vi "limitDecendantsTo1Level.vi"(8 "error in (no error)":errorcluster, 10 "hierarchy":string[][](array[string]), 11 "ClassLoader in":refnum<class "ClassLoader.lvclass">) -> (0 "error out":errorcluster, 2 "hierarchy out":string[][](array[string]), 3 "ClassLoader out":refnum<class "ClassLoader.lvclass">)   [LabVIEW 2020, in "JKI JSON Object Serialization.lvlib" / "OOP_Utility.lvlib" / "Reflection.lvclass"]
doc: "GCraftsman JSON Object Serialization Toolkit\nwww.GCraftsman.com\nCopyright (c) 2017, GCraftsman"
uses:
  Reflection.lvclass
  ClassLoader/ClassLoader.lvclass
  Reflection.lvclass/Reflection.ctl
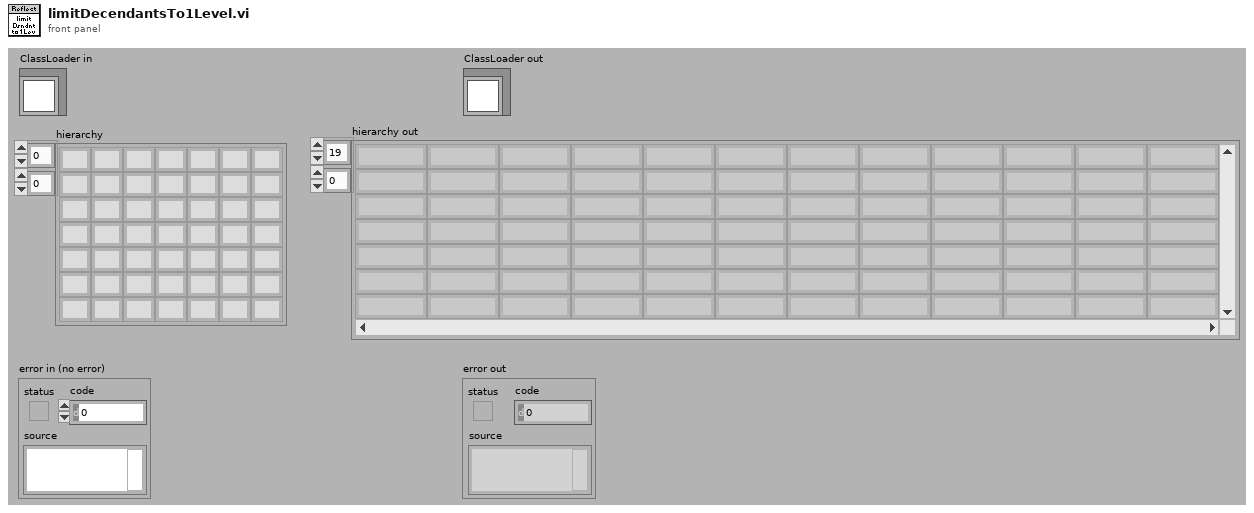
[diagram p1: front panel]
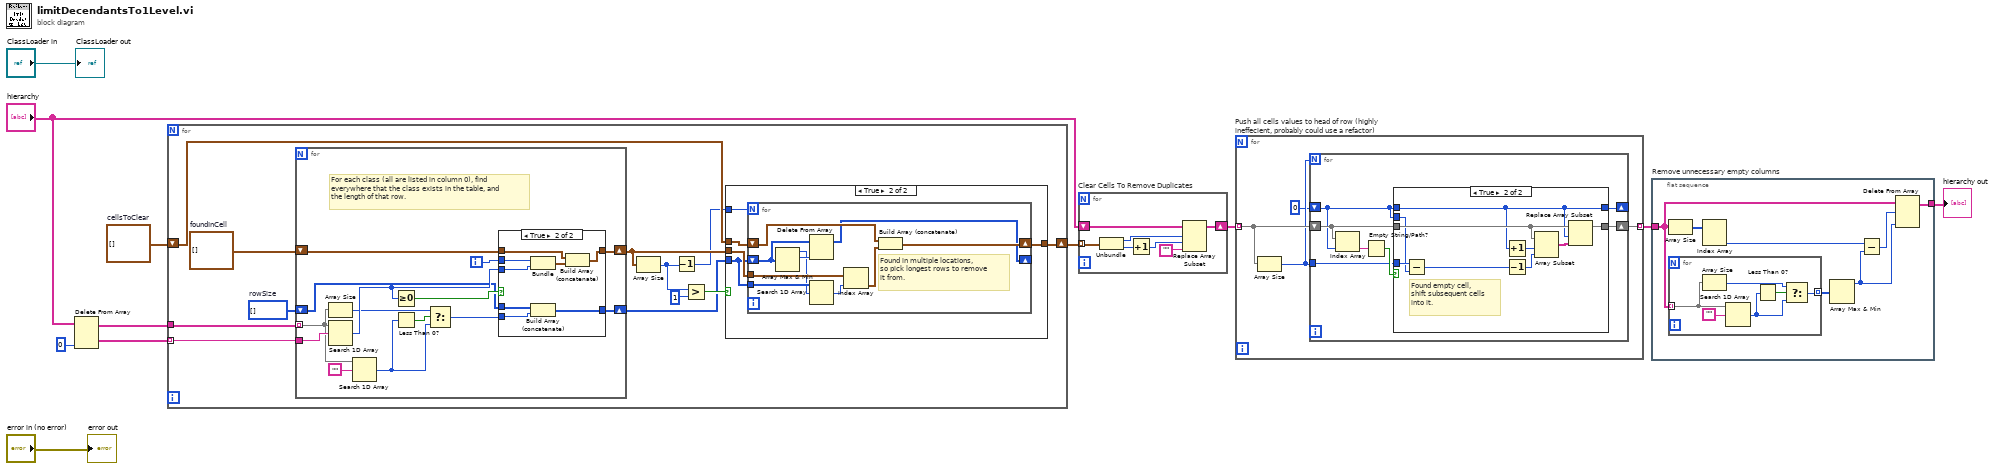
[diagram p0: block diagram]
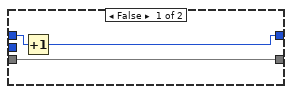
[diagram p2: hidden frame]
diagram:
  w8 = cluster{i32, "index of element":i32}[] []  # cellsToClear
  n1 = Delete From Array(array="hierarchy", index (col)=0 ("disabled index (col)")) -> (deleted portion=w4:string[], array with subset deleted=w5:string[][])  [unwired: 2 in]
  n2 = for {
    tunnel: w5 -> [w22]
    tunnel: w4 -> [w23] mode=indexing
    shift-right: [w15] -> w9
    shift-left: w8 -> [w14]
    w20 = i32[] []  # rowSize
    w21 = cluster{i32, "index of element":i32}[] []  # foundInCell
    n3 = for {
      tunnel: w23 -> [w52]
      tunnel: w22 -> [w43] mode=indexing
      shift-right: [w50] -> w16
      shift-left: w21 -> [w47]
      shift-right: [w46] -> w17
      shift-left: w20 -> [w45]
      i -> [w48]
      # "For each class (all are listed in column 0), find \neverywhere that the class exists in the table, and\nthe length of that row."
      n4 = Array Size(array=w43) -> (size(s)=w42:i32)
      n5 = Search 1D Array(1D array=w43, element=w52) -> (index of element=w49:i32)  [unwired: 1 in]
      n6 = Search 1D Array(1D array=w43, element="") -> (index of element=w41:i32)  [unwired: 1 in]
      n7 = Greater Or Equal To 0?(x=w49) -> (x >= 0?=w51:bool)
      n8 = Less Than 0?(x=w41) -> (x < 0?=w44:bool)
      n9 = Select(t=w42, s=w44, f=w41) -> (s? t:f=w40:i32)
      n10 = case shown="True" w51 {
        tunnel: w40 -> [_ w58]
        tunnel: [w55 w63] -> w50
        tunnel: w49 -> [_ w62]
        tunnel: w48 -> [_ w61]
        tunnel: w47 -> [w55 w59]
        tunnel: [w54 w57] -> w46
        tunnel: w45 -> [w54 w56]
        frame False {
        }
        frame True {
          n11 = Bundle(w61, "index of element"=w62) -> (w60:cluster{i32, "index of element":i32})  [unwired: 1 in]
          n12 = Build Array (concatenate)(w56, w58) -> (w57:i32[])
          n13 = Build Array (concatenate)(w59, w60) -> (w63:cluster{i32, "index of element":i32}[])
        }
      }
    }
    n14 = Array Size(array=w16) -> (size(s)=w13:i32)
    n15 = Decrement(x=w13) -> (x-1=w12:i32)
    n16 = Greater?(x=w13, y=1) -> (0:w18:bool)
    n17 = case shown="True" w18 {
      tunnel: w17 -> [_ w25]
      tunnel: w16 -> [_ w29]
      tunnel: [w24 w28] -> w15
      tunnel: w14 -> [w24 w27]
      tunnel: w12 -> [_ w26]
      frame False {
      }
      frame True {
        n18 = for {
          N: w26 -> [_]
          tunnel: w29 -> [w39]
          shift-right: [w37] -> w28
          shift-left: w27 -> [w36]
          shift-right: [w35] -> _
          shift-left: w25 -> [w32]
          tunnel: w25 -> [w33]
          # "Found in multiple locations,\nso pick longest rows to remove\nit from."
          n19 = Array Max & Min(array=w32) -> (max value=w31:i32, max index (indices)=w34:i32)  [unwired: 2 out]
          n20 = Delete From Array(array=w32, index=w34) -> (array with subset deleted=w35:i32[])  [unwired: 1 in, 1 out]
          n21 = Search 1D Array(1D array=w33, element=w31) -> (index of element=w30:i32)  [unwired: 1 in]
          n22 = Index Array(array=w39, index=w30) -> (element=w38:cluster{i32, "index of element":i32})
          n23 = Build Array (concatenate)(w36, w38) -> (w37:cluster{i32, "index of element":i32}[])
        }
      }
    }
  }
  n24 = for "Clear Cells To Remove Duplicates" {
    tunnel: w9 -> [w68] mode=indexing
    shift-right: [w64] -> w3
    shift-left: "hierarchy" -> [w70]
    n25 = Unbundle(w68) -> (w69:i32, "index of element"=w66:i32)
    n26 = Increment(x=w66) -> (x+1=w65:i32)
    n27 = Replace Array Subset(array=w70, new element="", index (row)=w69, index (col)=w65) -> (w64:string[][])
  }
  n28 = for "Push all cells values to head of row (highly ineffecient, probably could use a refactor)" {
    tunnel: w3 -> [w74] mode=indexing
    tunnel: [w73] -> w2 mode=indexing
    n29 = Array Size(array=w74) -> (size(s)=w72:i32)
    n30 = for {
      N: w72 -> [_]
      shift-right: [w78] -> w73
      shift-left: w74 -> [w80]
      tunnel: w72 -> [w76]
      shift-right: [w77] -> _
      shift-left: 0 -> [w75]
      n31 = Index Array(array=w80, index=w75) -> (element=w81:string)
      n32 = Empty String/Path?(string/path=w81) -> (empty?=w79:bool)
      n33 = case shown="True" w79 {
        tunnel: w80 -> [w84 w93]
        tunnel: w75 -> [w82 w85]
        tunnel: [w84 w91] -> w78
        tunnel: [w83 w85] -> w77
        tunnel: w76 -> [_ w89]
        tunnel: w75 -> [_ w88]
        frame False {
          n34 = Increment(x=w82) -> (x+1=w83:i32)
        }
        frame True {
          # "Found empty cell,\nshift subsequent cells\ninto it."
          n35 = Subtract(x=w89, y=w88) -> (x-y=w90:i32)
          n36 = Increment(x=w85) -> (x+1=w86:i32)
          n37 = Decrement(x=w90) -> (x-1=w87:i32)
          n38 = Array Subset(array=w93, index=w86, length=w87) -> (w92:string[])
          n39 = Replace Array Subset(array=w93, new element=w92, index=w85) -> (w91:string[])
        }
      }
    }
  }
  n40 = flat-sequence "Remove unnecessary empty columns" {
    tunnel: w2 -> [w99]
    tunnel: [w95] -> w1
    frame #0 {
      n41 = Array Size(array=w99) -> (size(s)=w98:i32[])
      n42 = for {
        tunnel: w99 -> [w103] mode=indexing
        tunnel: [w102] -> w100 mode=indexing
        n43 = Array Size(array=w103) -> (size(s)=w104:i32)
        n44 = Search 1D Array(1D array=w103, element="") -> (index of element=w101:i32)  [unwired: 1 in]
        n45 = Less Than 0?(x=w101) -> (x < 0?=w105:bool)
        n46 = Select(t=w104, s=w105, f=w101) -> (s? t:f=w102:i32)
      }
      n47 = Index Array(array=w98) -> (element #2=w97:i32)  [unwired: 2 in, 1 out]
      n48 = Array Max & Min(array=w100) -> (max value=w94:i32)  [unwired: 3 out]
      n49 = Subtract(x=w97, y=w94) -> (x-y=w96:i32)
      n50 = Delete From Array(array=w99, length=w96, index (col)=w94) -> (array with subset deleted=w95:string[][])  [unwired: 1 in, 1 out]
    }
  }
  "error out" <- "error in (no error)"
  "ClassLoader out" <- "ClassLoader in"
  "hierarchy out" <- w1
